vi "CTRE_PigeonIMU_SetParameter.vi"(6 "TareType":T1 items=["SetValue"=0, "AddOffset"=1, "MatchCompass"=2, "SetOffset"=255], 8 "error in (no error)":errorcluster, 9 "Value":dbl, 10 "Parameter":T2 items=["YawOffset"=160, "CompassOffset"=161, "BetaGain"=162, "Reserved163"=163, "GyroNoMotionCal"=164, "EnterCalibration"=165, "FusedHeadingOffset"=166, "StatusFrameRate"=169, "AccumZ"=170, "TempCompDisable"=171], 11 "Device ID (0)":u32) -> (0 "error out":errorcluster, 3 "Device ID Out":u8)   [LabVIEW 2016]
uses:
  <vilib>/Rock Robotics/WPI/ThirdParty/Sensors/Pigeon IMU/CTRE_PigeonIMU_Params.ctl
  <vilib>/Rock Robotics/WPI/ThirdParty/Sensors/Pigeon IMU/CTRE_PigeonIMU_TareType.ctl
  <vilib>/Rock Robotics/WPI/ThirdParty/Sensors/Pigeon IMU/CTRE_PigeonIMU_MessageIDs.ctl
  <vilib>/Rock Robotics/WPI/ThirdParty/Sensors/Pigeon IMU/CTRE_PigeonIMU_GlobalOps.ctl
  <vilib>/Rock Robotics/WPI/ThirdParty/Sensors/Pigeon IMU/CTRE_PigeonIMU_GlobalStatus.ctl
  <vilib>/Rock Robotics/WPI/ThirdParty/Sensors/Pigeon IMU/CTRE_PigeonIMU_PigeonState.ctl
  <vilib>/Rock Robotics/WPI/ThirdParty/Sensors/Pigeon IMU/CTRE_PigeonIMU_CalibrationMode.ctl
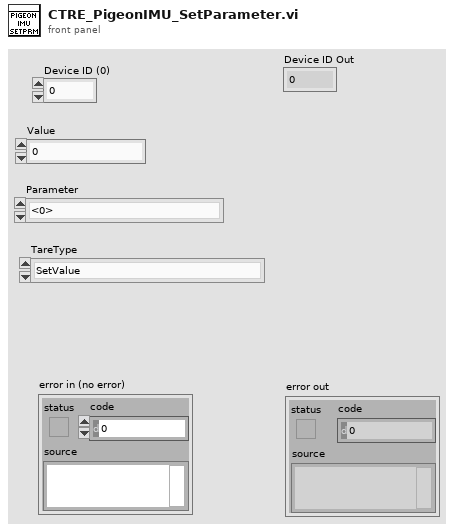
[diagram p1: front panel]
types:
  T1 = typedef "CTRE_PigeonIMU_TareType.ctl" = u8
  T2 = typedef "CTRE_PigeonIMU_Params.ctl" = u8
  T3 = typedef "CTRE_PigeonIMU_GlobalStatus.ctl" = cluster{"PigeonState":T4, "FusedHeading":cluster{"Heading":dbl, "Valid?":bool, "Fusing?":bool}, "YPR":cluster{"Yaw":dbl, "Pitch":dbl, "Roll":dbl}, "Compass":cluster{"Heading":dbl, "Magnitude":dbl, "Absolute Heading":dbl}, "Accelerometer":cluster{"Biased":cluster{"X":i16, "Y":i16, "Z":i16, "Norm":i16}, "Angles":cluster{"XZ Tilt":dbl, "YZ Tilt":dbl, "XY Tilt":dbl}}, "Magnetometer":cluster{"Raw":cluster{"X":i16, "Y":i16, "Z":i16}, "Biased":cluster{"X":i16, "Y":i16, "Z":i16}}, "Gyro":cluster{"X":dbl, "Y":dbl, "Z":dbl, "Norm":dbl}, "6D Quaternian":cluster{"W":dbl, "X":dbl, "Y":dbl, "Z":dbl}, "Temp. (C)":dbl, "UpTime":u32, "StartupStatus":cluster{"ResetCount":i32, "ResetFlags":i32, "FirmwareVersion":i32, "HasReset?":bool}, "Calibration":cluster{"CurrentMode":T5, "LastCalError":i32, "CalBooting?":bool}, "CAN Error":errorcluster, "AccumGyro":cluster{"X":dbl, "Y":dbl, "Z":dbl}}
  T4 = typedef "CTRE_PigeonIMU_PigeonState.ctl" = enum16{"NoComm", "Initializing", "Ready", "UserCalibration"}
  T5 = typedef "CTRE_PigeonIMU_CalibrationMode.ctl" = u16
  T6 = typedef "CTRE_PigeonIMU_GlobalOps.ctl" = enum16{"Read For Send", "Write Error", "Get All", "Set Control Frame Rate", "Set Enable Frame Rate", "Write After Receive Fused Heading", "Write After Receive YPR", "Write After Receive Status", "Write After Receive Raw Magnetomoter", "Write After Receive Biased Magnetometer", "Write After Receive Biased Accelerometer", "Write After Receive Gyro", "Write After Receive Acceleromter Angles", "Write After Receive Startup Status", "Write After Receive Compass", "Write After Receive Quaternian", "Write After Receive AccumGyro"}
  T7 = typedef "CTRE_PigeonIMU_MessageIDs.ctl" = u32
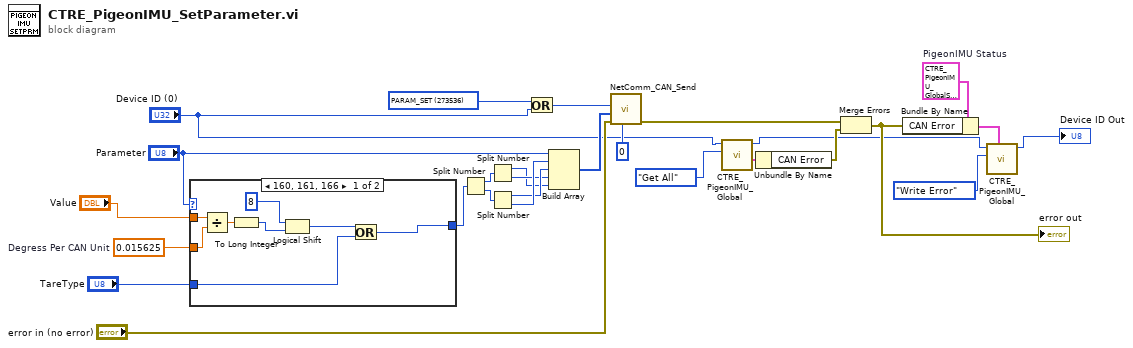
[diagram p0: block diagram]
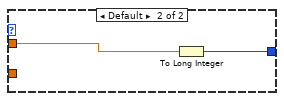
[diagram p2: hidden frame]
diagram:
  w5 = T3 {"PigeonState"=enum."NoComm", "FusedHeading"={"Heading"=0.0, "Valid?"=FALSE, "Fusing?"=FALSE}, "YPR"={"Yaw"=0.0, "Pitch"=0.0, "Roll"=0.0}, "Compass"={"Heading"=0.0, "Magnitude"=0.0, "Absolute Heading"=0.0}, "Accelerometer"={"Biased"={"X"=0, "Y"=0, "Z"=0, "Norm"=0}, "Angles"={"XZ Tilt"=0.0, "YZ Tilt"=0.0, "XY Tilt"=0.0}}, "Magnetometer"={"Raw"={"X"=0, "Y"=0, "Z"=0}, "Biased"={"X"=0, "Y"=0, "Z"=0}}, "Gyro"={"X"=0.0, "Y"=0.0, "Z"=0.0, "Norm"=0.0}, "6D Quaternian"={"W"=0.0, "X"=0.0, "Y"=0.0, "Z"=0.0}, "Temp. (C)"=0.0, "UpTime"=0, "StartupStatus"={"ResetCount"=0, "ResetFlags"=0, "FirmwareVersion"=0, "HasReset?"=FALSE}, "Calibration"={"CurrentMode"=0, "LastCalError"=0, "CalBooting?"=FALSE}, "CAN Error"={"status"=FALSE, "code"=0, "source"=""}, "AccumGyro"={"X"=0.0, "Y"=0.0, "Z"=0.0}}  # PigeonIMU Status
  w12 = T7 273536 items=["RAW_STATUS_2"=265280, "RAW_STATUS_4"=265408, "RAW_STATUS_6"=265536, "BIASED_STATUS_2"=269376, "BIASED_STATUS_4"=269504, "BIASED_STATUS_6"=269632, "COND_STATUS_1"=270336, "COND_STATUS_2"=270400, "COND_STATUS_3"=270464, "COND_STATUS_4"=270528, "COND_STATUS_5"=270592, "COND_STATUS_6"=270656, "COND_STATUS_7"=270720, "COND_STATUS_8"=270784, "COND_STATUS_9"=270848, "COND_STATUS_10"=270912, "CONTROL_1"=272384, "PARAM_REQUEST"=273408, "PARAM_RESPONSE"=273472, "PARAM_SET"=273536] ("MessageIDs")
  w1 = 0.015625  # Degress Per CAN Unit
  n1 = case shown="160, 161, 166" "Parameter" {
    tunnel: [w30 w37] -> w14
    tunnel: "Value" -> [w35 w36]
    tunnel: "TareType" -> [w31 _]
    tunnel: w1 -> [w34 _]
    frame 160, 161, 166 {
      n2 = Divide(x=w35, y=w34) -> (x/y=w33:dbl)
      n3 = To Long Integer(number=w33) -> (32bit integer=w28:i32)
      n4 = Logical Shift(y=8 ("x"), x=w28) -> (x << y=w32:i32)
      n5 = Or(x=w32, y=w31) -> (x .or. y?=w30:i32)
    }
    frame Default {
      n6 = To Long Integer(number=w36) -> (32bit integer=w37:i32)
    }
  }
  n7 = Split Number(x=w14) -> (hi(x)=w24:u16, lo(x)=w23:u16)
  n8 = Split Number(x=w24) -> (hi(x)=w18:u8, lo(x)=w19:u8)
  n9 = Split Number(x=w23) -> (hi(x)=w20:u8, lo(x)=w21:u8)
  n10 = Or(x=w12, y="Device ID (0)") -> (x .or. y?=w26:T7)
  n11 = Build Array("Parameter", w21, w20, w19, w18) -> (w27:T2[])
  n12 = call <vilib>:"NetComm_CAN_Send.vi"("Period (ms)"=0 ("milliseconds to wait"), "error in (no error)"="error in (no error)", "Data"=w27, "Message ID"=w26) -> ("error out"=w17:errorcluster)  [unwired: 7 in]
  n13 = call <vilib>:"CTRE_PigeonIMU_Global.vi"("Operation"=CTRE_PigeonIMU_GlobalOps."Get All" ("Enum"), "Device ID (0)"="Device ID (0)") -> ("Get All"=w9:T3, "Device ID Out"=w8:u8)  [unwired: 7 in, 1 out]
  n14 = Unbundle By Name(w9) -> ("CAN Error"=w15:errorcluster)
  n15 = Merge Errors(w17, w15) -> (w16:errorcluster)
  "error out" <- w16
  n16 = Bundle By Name(cluster=w5, "CAN Error"=w16) -> (w4:T3)
  n17 = call <vilib>:"CTRE_PigeonIMU_Global.vi"("Write After Receive"=w4, "Operation"=CTRE_PigeonIMU_GlobalOps."Write Error" ("Enum"), "Device ID (0)"=w8) -> ("Device ID Out"=→"Device ID Out":u8)  [unwired: 6 in, 2 out]
